vi "stageClose.vi"() -> (0 "error out":errorcluster)   [LabVIEW 2017]
uses:
  globalDevices.vi
  Stage/ximcLVx64/libximc.lvlib
panel:
  out "stage ids":cluster{"opaque pointer":u64, "id":i32}
  out "error in (no error)":errorcluster
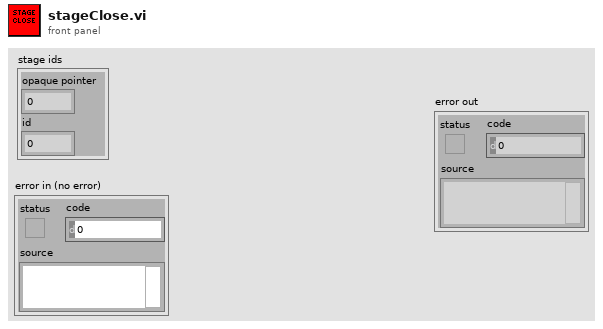
[diagram p1: front panel]
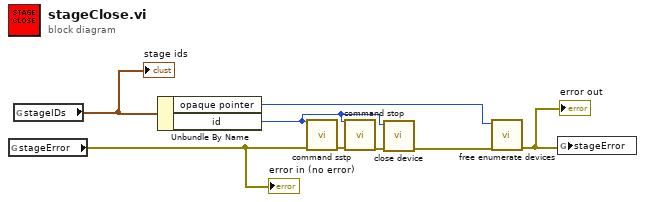
[diagram p0: block diagram]
diagram:
  n1 = global read "globalDevices.vi" "stageError"() -> (w2:errorcluster)
  "error in (no error)" <- w2
  n2 = global read "globalDevices.vi" "stageIDs"() -> (w3:cluster{"opaque pointer":u64, "id":i32})
  "stage ids" <- w3
  n3 = Unbundle By Name(w3) -> ("opaque pointer"=w8:u64, "id"=w6:i32)
  n4 = call "command sstp.vi"("error in (no error)"=w2, "id"=w6) -> ("error out"=w7:errorcluster)  [unwired: 8 in, 1 out]
  n5 = call "command stop.vi"("error in (no error)"=w7, "id"=w6) -> ("error out"=w5:errorcluster)  [unwired: 8 in, 1 out]
  n6 = call "close device.vi"("error in (no error)"=w5, "id"=w6) -> ("error out"=w4:errorcluster)  [unwired: 7 in, 2 out]
  n7 = call "free enumerate devices.vi"("error in (no error)"=w4, "device_enumeration"=w8) -> ("error out"=w1:errorcluster)  [unwired: 8 in, 1 out]
  "error out" <- w1
  n8 = global write "globalDevices.vi" "stageError"(w1) -> ()
